vi "Write X.vi"(8 "error in (no error)":errorcluster, 10 "X":dbl, 11 "JumpAbs in":refnum<class "JumpAbs.lvclass">) -> (0 "error out":errorcluster, 3 "JumpAbs out":refnum<class "JumpAbs.lvclass">)   [LabVIEW 2013, in "HardwareCharacterization.lvlib" / "JumpAbs.lvclass"]
uses:
  JumpAbs.lvclass
  JumpAbs.lvclass/JumpAbs.ctl
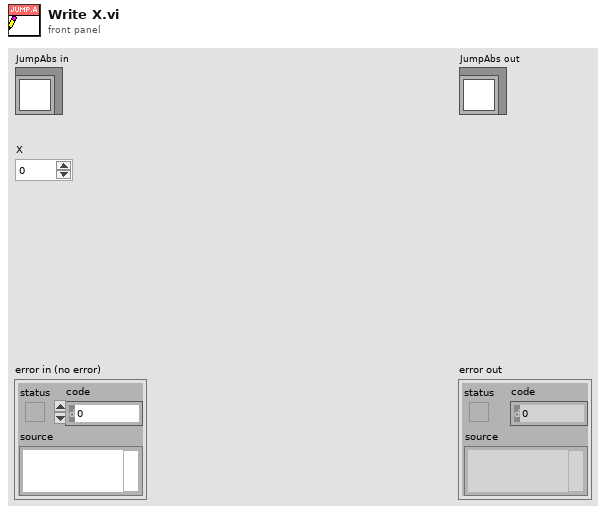
[diagram p1: front panel]
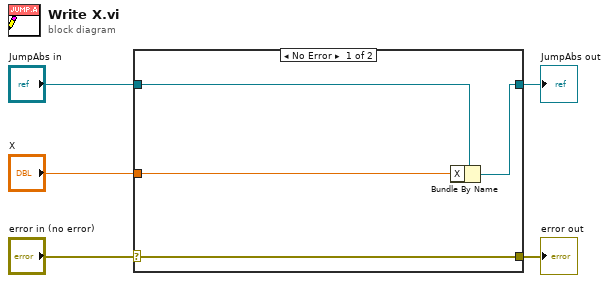
[diagram p0: block diagram]
diagram:
  n1 = case shown="No Error" "error in (no error)" {
    selector: "error in (no error)" -> [w9 w10]
    tunnel: [w9 w10] -> w4
    tunnel: [w7 w11] -> w2
    tunnel: "JumpAbs in" -> [w8 w11]
    tunnel: "X" -> [w6 _]
    frame No Error {
      n2 = Bundle By Name(cluster=w8, "X"=w6) -> (w7:refnum<class "JumpAbs.lvclass">)
    }
    frame Error {
    }
  }
  "error out" <- w4
  "JumpAbs out" <- w2
